vi "Save EEPROM To File.vi"(8 "error in (no error)":errorcluster, 11 "cFileName":string) -> (0 "error out":errorcluster, 2 "function return":u32, 3 "cFileName out":string)   [LabVIEW 2014, in "atmcd32d.lvlib"]
doc: "unsigned int WINAPI SaveEEPROMToFile(char * cFileName);"
uses:
  atmcd32d.lvlib
  atmcd32d.dll
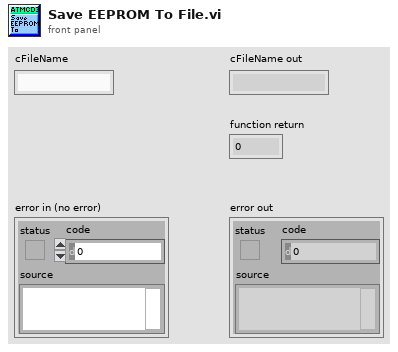
[diagram p1: front panel]
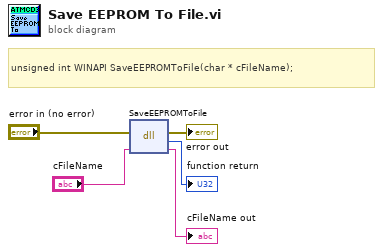
[diagram p0: block diagram]
diagram:
  # "unsigned int WINAPI SaveEEPROMToFile(char * cFileName);"
  n1 = dll-call lib="C:/Users/Bakir/Documents/Lambda2-Testing/lib/Andorlib/atmcd32d.*" fn="SaveEEPROMToFile"(error in="error in (no error)", "cFileName"="cFileName") -> (error out=→"error out":errorcluster, →"function return":u32, "cFileName"=→"cFileName out":string)  [unwired: 2 in, 1 out]
